vi "启动参数选择.vi"() -> (2 "check？":bool, 3 "启动参数输出":T1)   [LabVIEW 2016]
panel:
  in  "取消":bool
  in  "确定":bool
  in  "启动参数":T1
  # "请选择需要启动的参数"
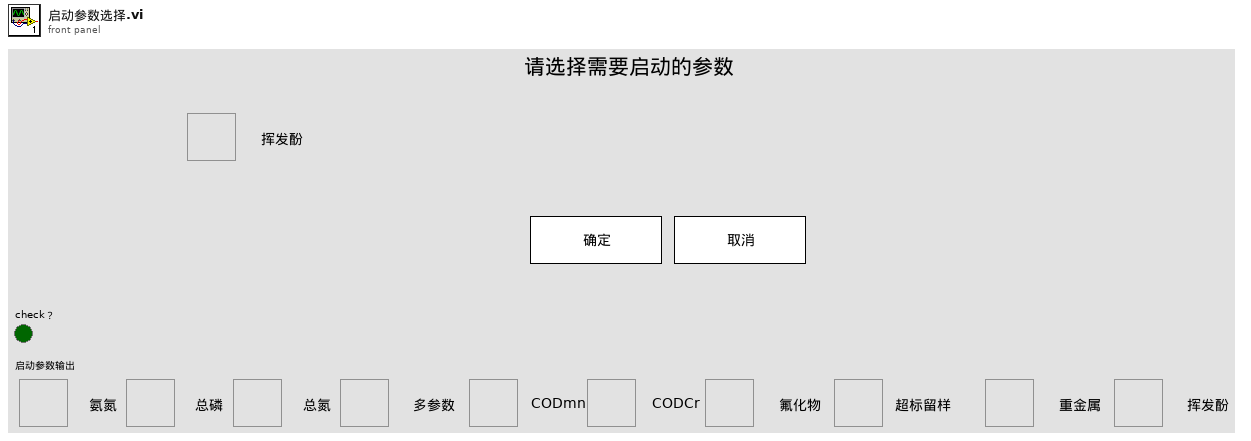
[diagram p1: front panel]
types:
  T1 = typedef "启动参数.ctl" = cluster{"氨氮":bool, "总磷":bool, "总氮":bool, "多参数":bool, "CODmn":bool, "CODCr":bool, "氟化物":bool, "超标留样":bool, "重金属":bool, "挥发酚":bool}
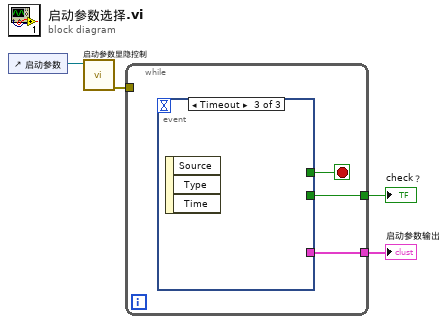
[diagram p0: block diagram]
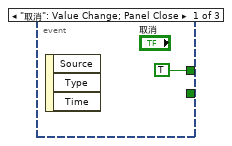
[diagram p2: hidden frame]
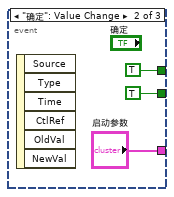
[diagram p3: hidden frame]
diagram:
  n1 = control-ref of="启动参数"() -> (w2:refnum<vi>)
  n2 = call "启动参数显隐控制.vi"("控件"=w2) -> ("error out"=w1:errorcluster)  [unwired: 10 in]
  n3 = while {
    tunnel: [w7] -> w3
    tunnel: [w5] -> w4
    tunnel: w1 -> [_]
    stop <- w6 stop-if-true
    n4 = event shown="[2] Timeout" {
      selector: _ -> [_ _ _]
      dyn-events: _ -> [_ _ _]
      timeout: _ -> [_ _ _]
      tunnel: [_ "启动参数" _] -> w7
      tunnel: [TRUE TRUE _] -> w6
      tunnel: [_ TRUE _] -> w5
      event "取消": Value Change; Panel Close {
        n5 = event-data() -> ()  [unwired: 1 in, 3 out]
      }
      event "确定": Value Change {
        n6 = event-data() -> ()  [unwired: 1 in, 6 out]
      }
      event Timeout {
        n7 = event-data() -> ()  [unwired: 1 in, 3 out]
      }
    }
  }
  "check？" <- w4
  "启动参数输出" <- w3
